vi "EPS_Test.vi"() -> ()   [LabVIEW 2019]
uses:
  Global1.vi
panel:
  out "data 2":string[][](array[string])
  out "data":string[][](array[string])
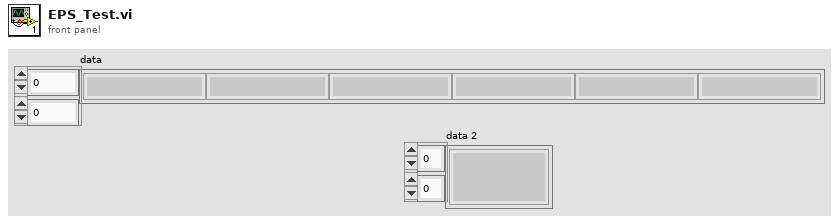
[diagram p1: front panel]
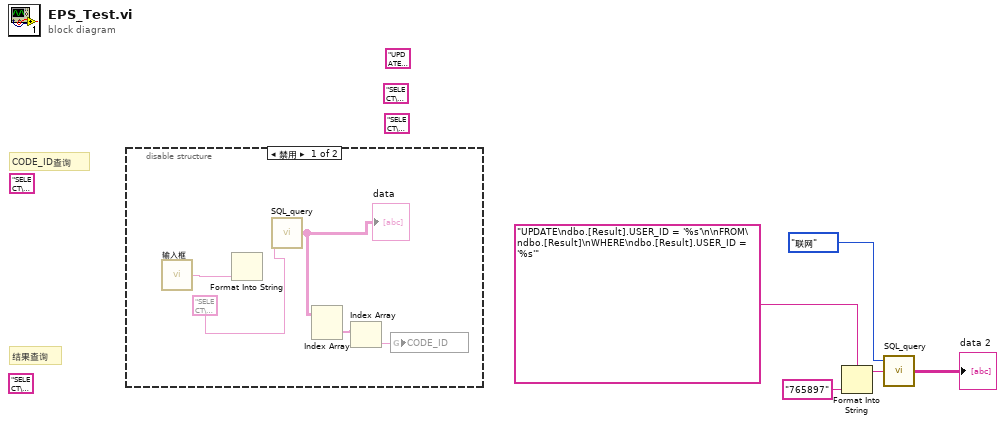
[diagram p0: block diagram]
diagram:
  (unwired) "SELECT\ndbo.[Result].RESULT_VALUE\nFROM\ndbo.[Result]\nWHERE\ndbo.[Result].CODE_ID = '%s'" ("格式字符串")
  (unwired) "SELECT\ndbo.[Code].CODE_ID,\ndbo.[Code].CODE_MAIN,\ndbo.[Code].PRODUCT_ID\n\nFROM\ndbo.[Code].CODE_MAIN = 'MACAU3001'" ("格式字符串")
  (unwired) "SELECT\n*\nFROM\ndbo.[Code]\nWHERE\ndbo.[Code].CODE_MAIN = 'MACAU3001'" ("格式字符串")
  (unwired) "UPDATE\ndbo.[Code]\nSET dbo.[Code].CODE_SENSOR = 'henglong'\nWHERE\ndbo.[Code].CODE_MAIN = 'MACAU3001'\n" ("格式字符串")
  (unwired) "SELECT\ndbo.[Code].CODE_ID\nFROM\ndbo.[Code]\nWHERE\ndbo.[Code].CODE_MAIN = '%s'" ("格式字符串")
  # "CODE_ID查询"
  # "结果查询"
  n1 = disable-structure shown="禁用" {
    frame Disabled {
      n2 = call "输入框.vi"() -> ("条形码输出"=w10:string)  [unwired: 1 in]
      n3 = Format Into String(w10) -> ()  [unwired: 3 in, 2 out]
      n4 = call "SQL_query.vi"("SQL query"="SELECT\ndbo.[Result].RESULT_VALUE,\ndbo.[Result].RESULT_ID\nFROM\ndbo.[Result]" ("格式字符串")) -> ("data"=w9:string[][])  [unwired: 2 in, 2 out]
      "data" <- w9
      n5 = Index Array(array=w9) -> (element=w8:string[])  [unwired: 2 in]
      n6 = Index Array(array=w8) -> (element=w7:string)  [unwired: 1 in]
      n7 = global write "Global1.vi" "CODE_ID"(w7) -> ()
    }
    frame Enabled {
    }
  }
  n8 = Format Into String(format string="UPDATE\ndbo.[Result].USER_ID = '%s'\n\nFROM\ndbo.[Result]\nWHERE\ndbo.[Result].USER_ID = '%s'" ("格式字符串"), "765897" ("输入 1")) -> (resulting string=w5:string)  [unwired: 2 in, 1 out]
  n9 = call "SQL_query.vi"("SQL query"=w5, "联机模式"=enum16{"单机", "联网"}."联网") -> ("data"=→"data 2":string[][])  [unwired: 1 in, 2 out]
